vi "SM correction ver2.vi"(0 "V in x":dbl, 1 "nm in":dbl, 2 "V in y":dbl, 3 "V x initial":dbl, 4 "Volts/pixel":dbl, 5 "V y initial":dbl, 8 "Array":dbl[][](array[numeric])) -> (6 "V out x":dbl[](array[numeric]), 7 "V out y":dbl[](array[numeric]))   [LabVIEW 2010]
uses:
  <vilib>/measure/NI_MABase.lvlib
panel:
  out "V offset y":dbl
  out "V offset x":dbl
  # "nmi"
  # "nmf"
  # "deltax"
  # "deltay"
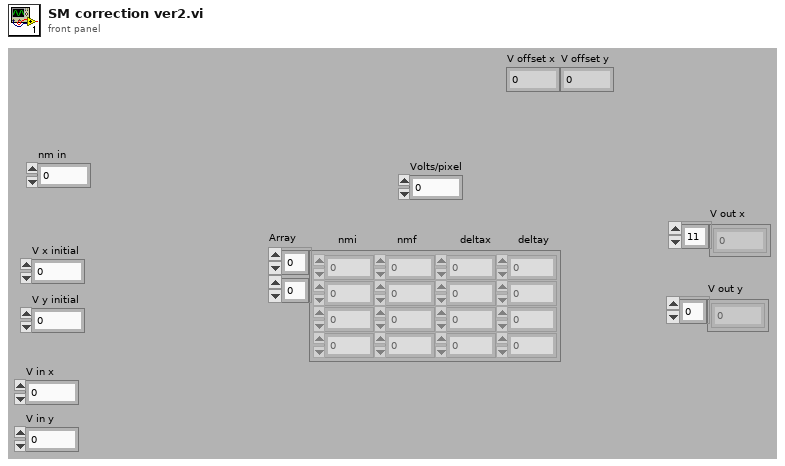
[diagram p1: front panel]
types:
  T1 = enum16{"Sine Wave", "Triangle Wave", "Square Wave", "Sawtooth Wave"}
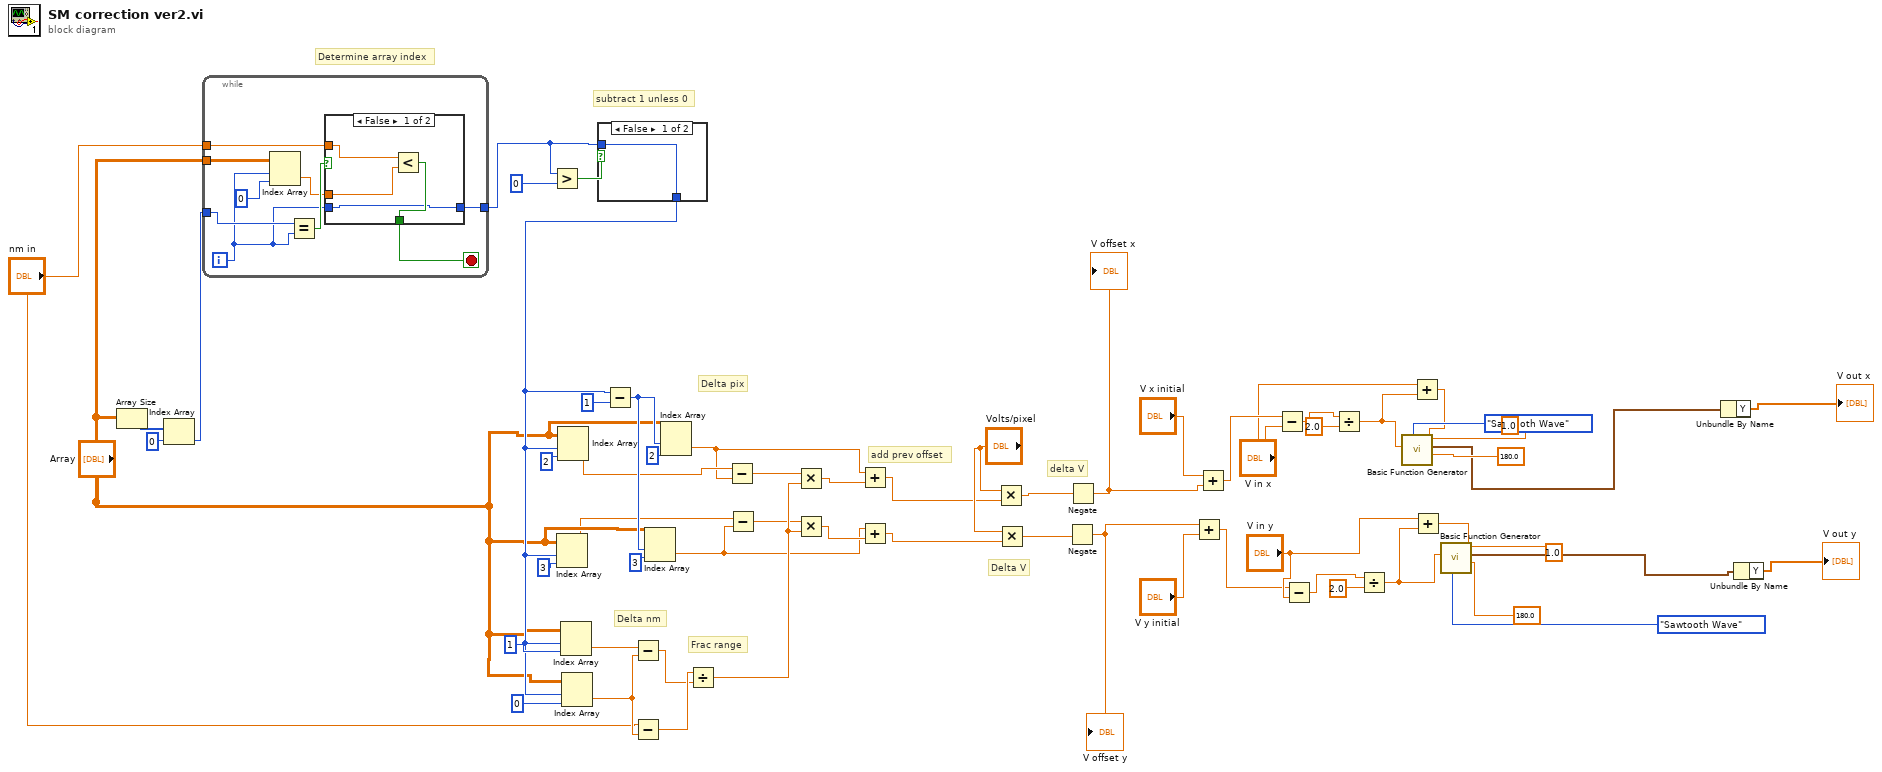
[diagram p0: block diagram]
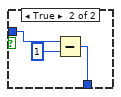
[diagram p2: hidden frame]
diagram:
  # "delta V"
  # "add prev offset"
  # "Frac range"
  # "subtract 1 unless 0"
  # "Determine array index"
  # "Delta nm"
  # "Delta V"
  # "Delta pix"
  n1 = Array Size(array="Array") -> (size(s)=w54:i32[])
  n2 = Index Array(array=w54, index=0) -> (element=w52:i32)
  n3 = while {
    tunnel: w52 -> [w68]
    tunnel: "nm in" -> [w65]
    tunnel: [w67] -> w48
    tunnel: "Array" -> [w63]
    i -> [w62]
    stop <- w66 stop-if-true
    n4 = Index Array(array=w63, index (row)=w62, index (col)=0 ("disabled index (col)")) -> (element=w64:dbl)
    n5 = Equal?(x=w68, y=w62) -> (x = y?=w69:bool)
    n6 = case shown="False" w69 {
      selector: w69 -> [_ w75]
      tunnel: w62 -> [w71 w76]
      tunnel: [w71 w76] -> w67
      tunnel: [w72 w75] -> w66
      tunnel: w65 -> [w74 _]
      tunnel: w64 -> [w73 _]
      frame False {
        n7 = Less?(x=w74, y=w73) -> (x < y?=w72:bool)
      }
      frame True {
      }
    }
  }
  n8 = Greater?(x=w48, y=0) -> (0:w49:bool)
  n9 = case shown="False" w49 {
    tunnel: w48 -> [w77 w80]
    tunnel: [w77 w78] -> w45
    frame False {
    }
    frame True {
      n10 = Subtract(x=w80, y=1) -> (x-y=w78:i32)
    }
  }
  n11 = Index Array(array="Array", index (row)=w45, index (col)=3 ("index")) -> (element=w38:dbl)
  n12 = Index Array(array="Array", index (row)=w45, index (col)=2 ("index")) -> (element=w39:dbl)
  n13 = Index Array(array="Array", index (row)=w45, index (col)=1 ("index")) -> (element=w60:dbl)
  n14 = Index Array(array="Array", index (row)=w45, index (col)=0 ("index")) -> (element=w55:dbl)
  n15 = Subtract(x=w45, y=1) -> (x-y=w43:i32)
  n16 = Subtract(x=w60, y=w55) -> (x-y=w46:dbl)
  n17 = Subtract(x="nm in", y=w55) -> (x-y=w47:dbl)
  n18 = Index Array(array="Array", index (row)=w43, index (col)=3) -> (element=w32:dbl)
  n19 = Index Array(array="Array", index (row)=w43, index (col)=2) -> (element=w31:dbl)
  n20 = Divide(x=w47, y=w46) -> (x/y=w37:dbl)
  n21 = Subtract(x=w39, y=w31) -> (x-y=w36:dbl)
  n22 = Subtract(x=w38, y=w32) -> (x-y=w35:dbl)
  n23 = Multiply(x=w36, y=w37) -> (x*y=w34:dbl)
  n24 = Multiply(x=w35, y=w37) -> (x*y=w33:dbl)
  n25 = Add(x=w31, y=w34) -> (x+y=w30:dbl)
  n26 = Add(x=w32, y=w33) -> (x+y=w29:dbl)
  n27 = Multiply(x="Volts/pixel", y=w30) -> (x*y=w25:dbl)
  n28 = Multiply(x="Volts/pixel", y=w29) -> (x*y=w21:dbl)
  n29 = Negate(x=w21) -> (-x=w19:dbl)
  "V offset y" <- w19
  n30 = Negate(x=w25) -> (-x=w20:dbl)
  "V offset x" <- w20
  n31 = Add(x=w19, y="V y initial") -> (x+y=w5:dbl)
  n32 = Add(x="V x initial", y=w20) -> (x+y=w18:dbl)
  n33 = Subtract(x=w18, y="V in x") -> (x-y=w16:dbl)
  n34 = Subtract(x=w5, y="V in y") -> (x-y=w10:dbl)
  n35 = Divide(x=w16, y=2.0) -> (x/y=w13:dbl)
  n36 = Divide(x=w10, y=2.0) -> (x/y=w8:dbl)
  n37 = Add(x="V in x", y=w13) -> (x+y=w12:dbl)
  n38 = call <vilib>:"Basic Function Generator.vi"("offset"=w12, "signal type"=T1."Sawtooth Wave", "phase"=180.0, "amplitude"=w13, "frequency"=1.0) -> ("signal out"=w4:waveform(dbl))  [unwired: 4 in, 2 out]
  n39 = Add(x="V in y", y=w8) -> (x+y=w7:dbl)
  n40 = call <vilib>:"Basic Function Generator.vi"("offset"=w7, "signal type"=T1."Sawtooth Wave", "phase"=180.0, "amplitude"=w8, "frequency"=1.0) -> ("signal out"=w3:waveform(dbl))  [unwired: 4 in, 2 out]
  n41 = Unbundle By Name(w4) -> ("Y"=→"V out x":dbl[])
  n42 = Unbundle By Name(w3) -> ("Y"=→"V out y":dbl[])
